vi "inc.dec.timeframe.vi"(9 "inc (T)":bool, 10 "Step Size":enum32{"Monthly", "Yearly"}(ring), 11 "Plot End":timestamp) -> (3 "time stamp":timestamp)   [LabVIEW 2024]
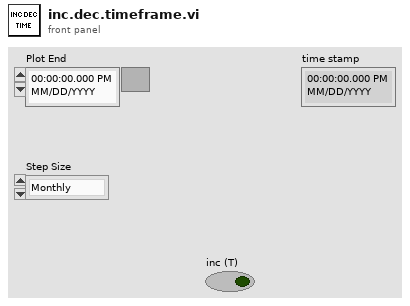
[diagram p1: front panel]
types:
  T1 = typedef "LVDateTimeRec.ctl" = cluster{"fractional second":dbl, "second":i32, "minute":i32, "hour":i32, "day of month":i32, "month":i32, "year":i32, "day of week":i32, "day of year":i32, "DST":i32}
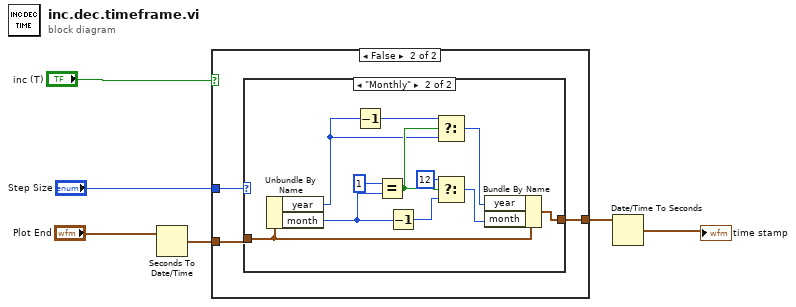
[diagram p0: block diagram]
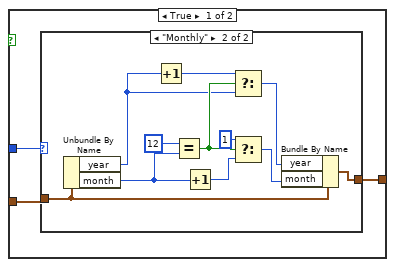
[diagram p2: hidden frame]
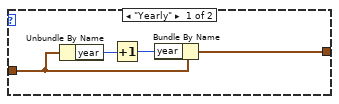
[diagram p3: hidden frame]
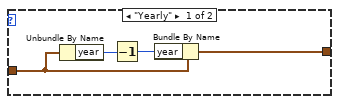
[diagram p4: hidden frame]
diagram:
  n1 = Seconds To Date/Time(time stamp (now)="Plot End") -> (date time rec=w3:T1)  [unwired: 1 in]
  n2 = case shown="False" "inc (T)" {
    tunnel: "Step Size" -> [w9 w27]
    tunnel: w3 -> [w8 w26]
    tunnel: [w7 w25] -> w2
    frame True {
      n3 = case shown="\"Monthly\"" w9 {
        tunnel: w8 -> [w11 w24]
        tunnel: [w10 w23] -> w7
        frame "Yearly" {
          n4 = Unbundle By Name(w11) -> ("year"=w13:i32)
          n5 = Increment(x=w13) -> (x+1=w12:i32)
          n6 = Bundle By Name(cluster=w11, "year"=w12) -> (w10:T1)
        }
        frame "Monthly" {
          n7 = Unbundle By Name(w24) -> ("year"=w15:i32, "month"=w22:i32)
          n8 = Increment(x=w15) -> (x+1=w14:i32)
          n9 = Equal?(x=12, y=w22) -> (x = y?=w16:bool)
          n10 = Increment(x=w22) -> (x+1=w20:i32)
          n11 = Select(t=w14, s=w16, f=w15) -> (s? t:f=w17:i32)
          n12 = Select(t=1, s=w16, f=w20) -> (s? t:f=w18:i32)
          n13 = Bundle By Name(cluster=w24, "year"=w17, "month"=w18) -> (w23:T1)
        }
      }
    }
    frame False {
      n14 = case shown="\"Monthly\"" w27 {
        tunnel: w26 -> [w29 w42]
        tunnel: [w28 w41] -> w25
        frame "Yearly" {
          n15 = Unbundle By Name(w29) -> ("year"=w31:i32)
          n16 = Decrement(x=w31) -> (x-1=w30:i32)
          n17 = Bundle By Name(cluster=w29, "year"=w30) -> (w28:T1)
        }
        frame "Monthly" {
          n18 = Unbundle By Name(w42) -> ("year"=w33:i32, "month"=w40:i32)
          n19 = Decrement(x=w33) -> (x-1=w32:i32)
          n20 = Equal?(x=1, y=w40) -> (x = y?=w35:bool)
          n21 = Decrement(x=w40) -> (x-1=w38:i32)
          n22 = Select(t=w32, s=w35, f=w33) -> (s? t:f=w34:i32)
          n23 = Select(t=12, s=w35, f=w38) -> (s? t:f=w36:i32)
          n24 = Bundle By Name(cluster=w42, "year"=w34, "month"=w36) -> (w41:T1)
        }
      }
    }
  }
  n25 = Date/Time To Seconds(2:w2) -> (0:→"time stamp":timestamp)  [unwired: 1 in]
